vi "sub_apt_setblash.vi"(8 "错误输入（无错误）":errorcluster, 11 "引用":refnum<k7>) -> (0 "错误输出":errorcluster, 3 "引用输出":refnum<k7>)   [LabVIEW 2015]
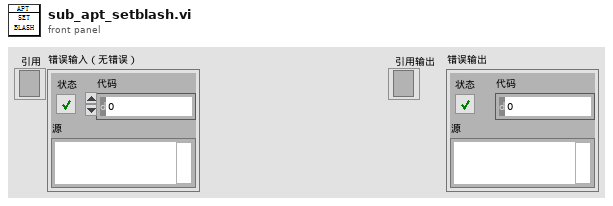
[diagram p1: front panel]
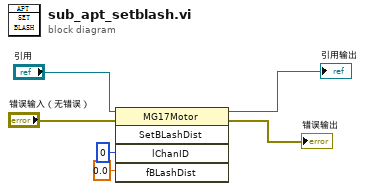
[diagram p0: block diagram]
diagram:
  n1 = invoke class="MG17Motor" method="SetBLashDist"(reference="引用", error in="错误输入（无错误）", "lChanID"=0, "fBLashDist"=sgl 0.0) -> (reference out=→"引用输出":refnum<k7>, error out=→"错误输出":errorcluster)  [unwired: 1 in, 3 out]
